vi "Distance and Turn Conversion.vi"(6 "Turn?":bool, 8 "Inches/Degrees Left":dbl, 9 "CAN Talon SRX Ref Left In":T1={"DeviceStatus"={"status"=FALSE, "code"=0, "source"=""}, "Type"=enum."PWM", "PWM"={"PWM Channel"=enum."PWM 1", "DeadBand"={"Name"="", "maxPositivePwm"=0, "minPositivePwm"=0, "centerPwm"=0, "maxNegativePwm"=0, "minNegativePwm"=0, "angularRange"=0}}, "CAN"={"Device Number"=0, "SetOutput VI Ref"=variant(enum8{"Percent VBus", "Current", "Speed", "Position", "Voltage"} enum."Percent VBus"), "GetOutput VI Ref"=variant(refnum<k1> refnum), "Enable VI Ref"=variant(dbl 12.0), "Disable VI Ref"=variant(enum8{"Percent VBus", "Speed", "Position", "Slave", "Unchanged / Invalid", "Voltage Compensation", "Current", "Motion Profile"} enum."Percent VBus"), "Data"=variant}, "Invert"=FALSE}, 10 "Inches/Degrees Right":dbl, 11 "CAN Talon SRX Ref Right In":T1={"DeviceStatus"={"status"=FALSE, "code"=0, "source"=""}, "Type"=enum."PWM", "PWM"={"PWM Channel"=enum."PWM 1", "DeadBand"={"Name"="", "maxPositivePwm"=0, "minPositivePwm"=0, "centerPwm"=0, "maxNegativePwm"=0, "minNegativePwm"=0, "angularRange"=0}}, "CAN"={"Device Number"=0, "SetOutput VI Ref"=variant(enum8{"Percent VBus", "Current", "Speed", "Position", "Voltage"} enum."Percent VBus"), "GetOutput VI Ref"=variant(refnum<k1> refnum), "Enable VI Ref"=variant(dbl 12.0), "Disable VI Ref"=variant(enum8{"Percent VBus", "Speed", "Position", "Slave", "Unchanged / Invalid", "Voltage Compensation", "Current", "Motion Profile"} enum."Percent VBus"), "Data"=variant}, "Invert"=FALSE}) -> (1 "CAN Talon SRX Ref Left Out":T1={"DeviceStatus"={"status"=FALSE, "code"=0, "source"=""}, "Type"=enum."PWM", "PWM"={"PWM Channel"=enum."Invalid", "DeadBand"={"Name"="", "maxPositivePwm"=0, "minPositivePwm"=0, "centerPwm"=0, "maxNegativePwm"=0, "minNegativePwm"=0, "angularRange"=0}}, "CAN"={"Device Number"=0, "SetOutput VI Ref"=variant, "GetOutput VI Ref"=variant, "Enable VI Ref"=variant, "Disable VI Ref"=variant, "Data"=variant}, "Invert"=FALSE}, 3 "CAN Talon SRX Ref Right Out":T1={"DeviceStatus"={"status"=FALSE, "code"=0, "source"=""}, "Type"=enum."PWM", "PWM"={"PWM Channel"=enum."Invalid", "DeadBand"={"Name"="", "maxPositivePwm"=0, "minPositivePwm"=0, "centerPwm"=0, "maxNegativePwm"=0, "minNegativePwm"=0, "angularRange"=0}}, "CAN"={"Device Number"=0, "SetOutput VI Ref"=variant, "GetOutput VI Ref"=variant, "Enable VI Ref"=variant, "Disable VI Ref"=variant, "Data"=variant}, "Invert"=FALSE}, 4 "Both In Range":bool)   [LabVIEW 2016]
uses:
  <vilib>/Rock Robotics/WPI/MotorControl/WPI_MotorControlDeviceRef.ctl
  <vilib>/Rock Robotics/WPI/MotorControl/WPI_MotorControlType.ctl
  <vilib>/Rock Robotics/SystemInterfaces/DIO/FPGA_DIOPWMChannel.ctl
  <vilib>/Rock Robotics/WPI/PWM/WPI_PWMDeadband.ctl
  <vilib>/Rock Robotics/WPI/ThirdParty/CanMotor/TalonSRX/WPI_CANTalonSRX_APIControlMode.ctl
panel:
  out "Right Rotations":dbl
  out "Left Rotations":dbl
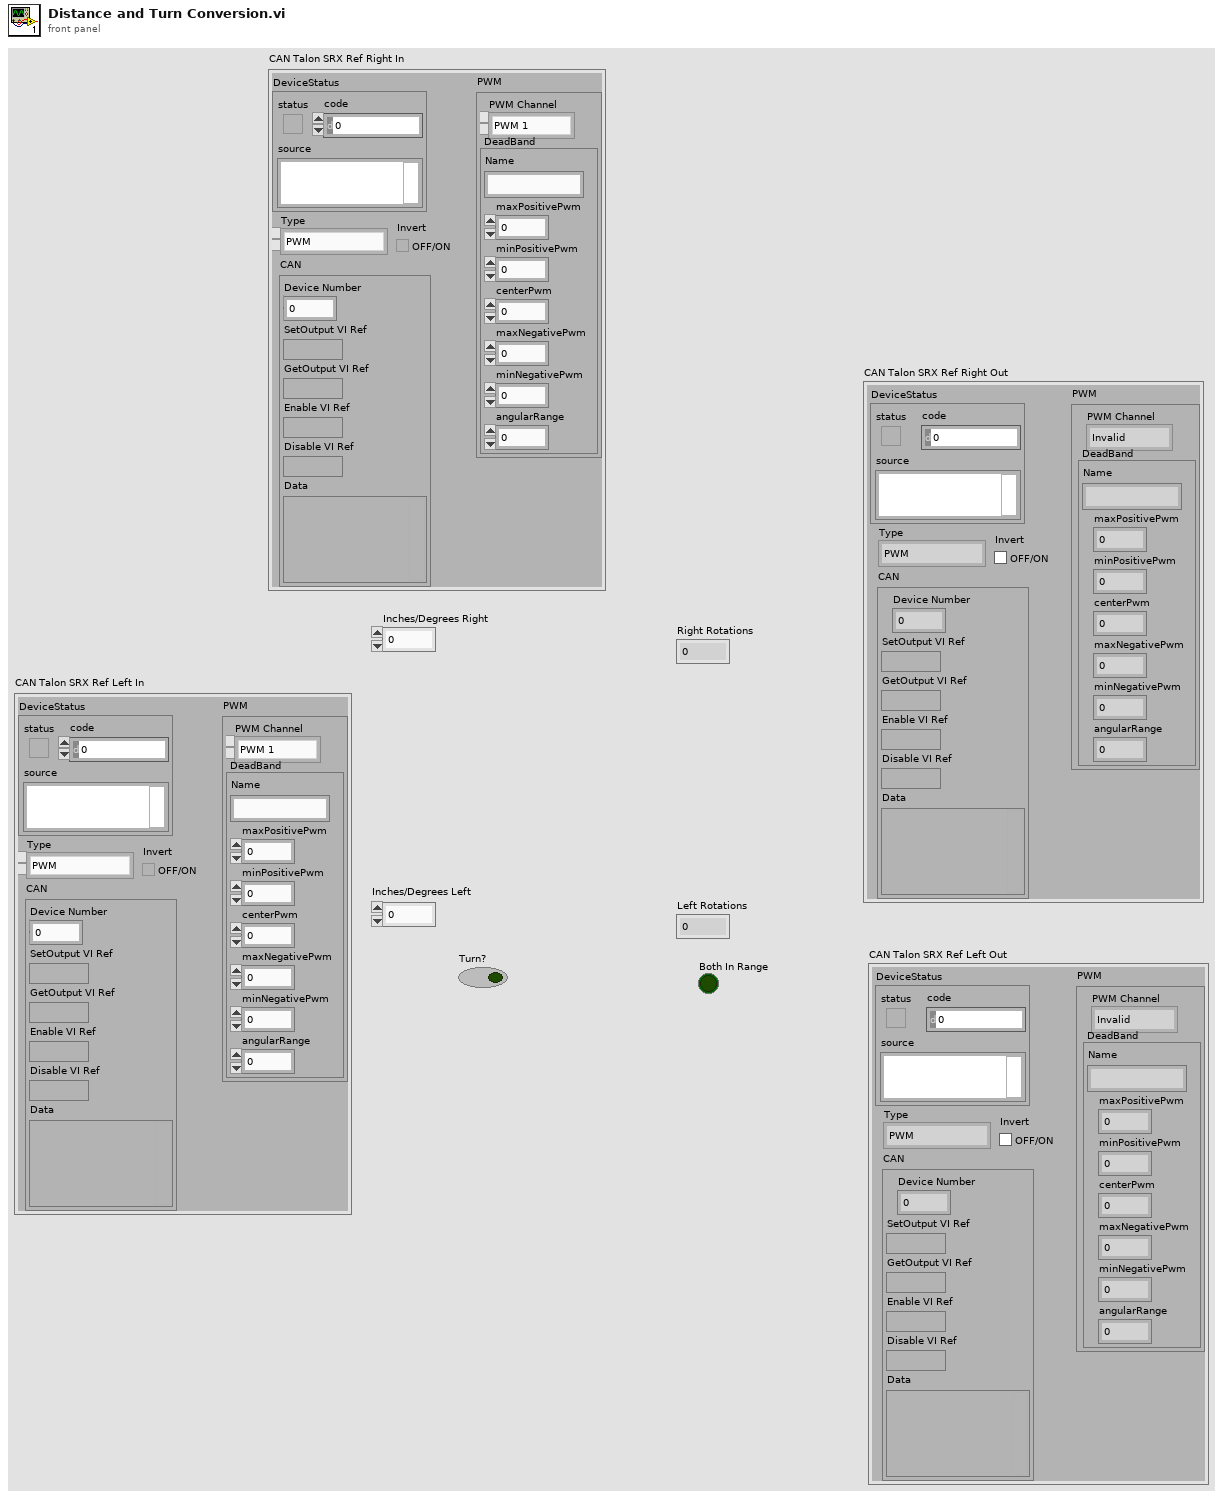
[diagram p1: front panel]
types:
  T1 = typedef "WPI_MotorControlDeviceRef.ctl" = cluster{"DeviceStatus":errorcluster, "Type":T2, "PWM":cluster{"PWM Channel":T3, "DeadBand":T4}, "CAN":cluster{"Device Number":u8, "SetOutput VI Ref":variant, "GetOutput VI Ref":variant, "Enable VI Ref":variant, "Disable VI Ref":variant, "Data":variant}, "Invert":bool}
  T2 = typedef "WPI_MotorControlType.ctl" = enum16{"PWM", "CAN"}
  T3 = typedef "FPGA_DIOPWMChannel.ctl" = enum8{"PWM 0", "PWM 1", "PWM 2", "PWM 3", "PWM 4", "PWM 5", "PWM 6", "PWM 7", "PWM 8", "PWM 9", "PWM MXP 0", "PWM MXP 1", "PWM MXP 2", "PWM MXP 3", "PWM MXP 4", "PWM MXP 5", "PWM MXP 6", "PWM MXP 7", "PWM MXP 8", "PWM MXP 9", "Invalid"}
  T4 = typedef "WPI_PWMDeadband.ctl" = cluster{"Name":string, "maxPositivePwm":i32, "minPositivePwm":i32, "centerPwm":i32, "maxNegativePwm":i32, "minNegativePwm":i32, "angularRange":u16}
  T5 = typedef "WPI_CANTalonSRX_APIControlMode.ctl" = enum8{"Percent VBus", "Speed", "Position", "Slave", "Unchanged / Invalid", "Voltage Compensation", "Current", "Motion Profile", "Motion Magic"}
  T6 = typedef "WPI_CANTalonSRX_GlobalStatus.ctl" = cluster{"Applied Throttle":dbl, "Module Enabled":bool, "CAN Error":errorcluster, "Closed Loop Error":dbl, "Forward Limit Switch Closed":bool, "Reverse Limit Switch Closed":bool, "Sensor Position":dbl, "Sensor Velocity":dbl, "Current":dbl, "Sticky Fault - Over Temp":bool, "Sticky Fault - Under Voltage":bool, "Sticky Fault - Forward Limit":bool, "Sticky Fault - Reverse Limit":bool, "Sticky Fault - Forward Soft Limit":bool, "Sticky Fault - Reverse Soft Limit":bool, "Brake is Enabled":bool, "Encoder Position":dbl, "Encoder Velocity":dbl, "Encoder Index Count":dbl, "Encoder A Pin State":bool, "Encoder B Pin State":bool, "Encoder Index Pin State":bool, "Analog In":dbl, "Analog In Velocity":dbl, "Temperature (C)":dbl, "Battery Voltage":dbl, "Control 5 Is Supported":bool, "Current Profile Slot Select":dbl, "Pos Div 8":bool, "Vel Div 4":bool, "Pulse Width Position":i32, "Pulse Width Velocity":i32, "Pulse Width Rise To Rise (us)":i32, "Pulse Width Rise To Fall (us)":i32, "Mot Prof Active Is Under Run":bool, "Mot Prof Active Has Under Run":bool, "Mot Prof Active Is Last":bool, "Mot Prof Active Velocity Only":bool, "Mot Prof Active Is Valid":bool, "Mot Prof Buffer Is Full":bool, "Mot Prof Active Profile Slot Select":i32, "Mot Prof NextID":i32, "Mot Prof Count":i32, "Mot Prof Active Velocity":dbl, "Mot Prof Active Position":dbl, "Mot Prof Output Enable":i32}
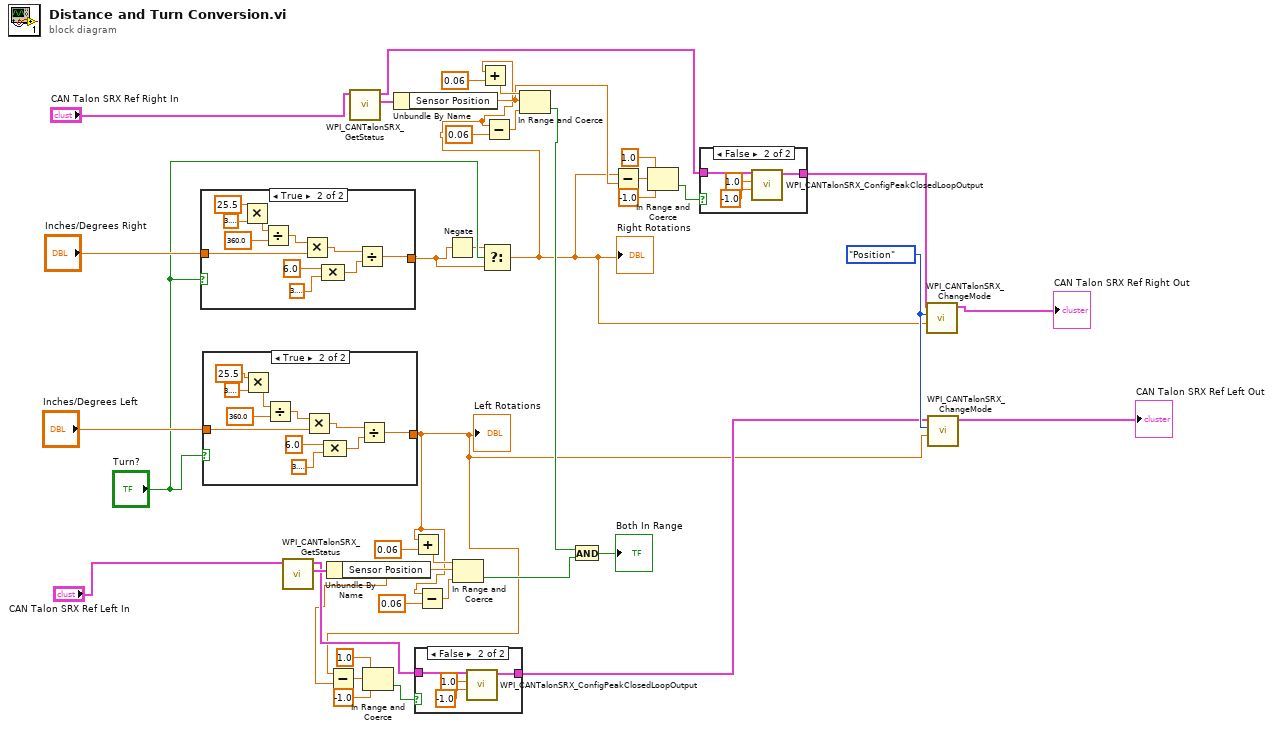
[diagram p0: block diagram]
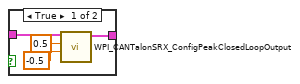
[diagram p2: hidden frame]
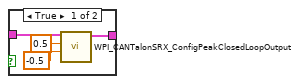
[diagram p3: hidden frame]
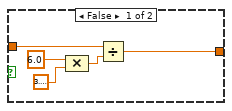
[diagram p4: hidden frame]
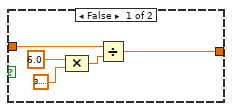
[diagram p5: hidden frame]
diagram:
  w7 = WPI_CANTalonSRX_APIControlMode."Position" ("Control Mode")
  n1 = case shown="True" "Turn?" {
    tunnel: "Inches/Degrees Right" -> [w42 w53]
    tunnel: [w40 w48] -> w35
    frame False {
      n2 = Compound Arithmetic op=MULTIPLY(6.0 ("value"), 3.141592653589793) -> (w41:dbl)
      n3 = Divide(x=w42, y=w41) -> (x/y=w40:dbl)
    }
    frame True {
      n4 = Multiply(x=25.5, y=3.141592653589793) -> (x*y=w46:dbl)
      n5 = Divide(x=w46, y=360.0) -> (x/y=w54:dbl)
      n6 = Multiply(x=w54, y=w53) -> (x*y=w49:dbl)
      n7 = Compound Arithmetic op=MULTIPLY(6.0 ("value"), 3.141592653589793) -> (w50:dbl)
      n8 = Divide(x=w49, y=w50) -> (x/y=w48:dbl)
    }
  }
  n9 = case shown="True" "Turn?" {
    tunnel: "Inches/Degrees Left" -> [w58 w69]
    tunnel: [w56 w64] -> w1
    frame False {
      n10 = Compound Arithmetic op=MULTIPLY(6.0 ("value"), 3.141592653589793) -> (w57:dbl)
      n11 = Divide(x=w58, y=w57) -> (x/y=w56:dbl)
    }
    frame True {
      n12 = Multiply(x=25.5, y=3.141592653589793) -> (x*y=w62:dbl)
      n13 = Divide(x=w62, y=360.0) -> (x/y=w70:dbl)
      n14 = Multiply(x=w70, y=w69) -> (x*y=w65:dbl)
      n15 = Compound Arithmetic op=MULTIPLY(6.0 ("value"), 3.141592653589793) -> (w66:dbl)
      n16 = Divide(x=w65, y=w66) -> (x/y=w64:dbl)
    }
  }
  "Left Rotations" <- w1
  n17 = call <vilib>:"WPI_CANTalonSRX_GetStatus.vi"("CAN Talon SRX Ref"="CAN Talon SRX Ref Left In") -> ("Talon SRX Status"=w28:T6, "CAN Talon SRX Ref"=w15:T1)  [unwired: 8 in, 1 out]
  n18 = Unbundle By Name(w28) -> ("Sensor Position"=w14:dbl)
  n19 = Subtract(x=w1, y=w14) -> (x-y=w19:dbl)
  n20 = call <vilib>:"WPI_CANTalonSRX_GetStatus.vi"("CAN Talon SRX Ref"="CAN Talon SRX Ref Right In") -> ("Talon SRX Status"=w34:T6, "CAN Talon SRX Ref"=w8:T1)  [unwired: 8 in, 1 out]
  n21 = In Range and Coerce(upper limit=1.0, x=w19, lower limit=-1.0) -> (In Range?=w16:bool)  [unwired: 1 out]
  n22 = Unbundle By Name(w34) -> ("Sensor Position"=w9:dbl)
  n23 = Add(x=w1, y=0.06) -> (x+y=w27:dbl)
  n24 = case shown="False" w16 {
    tunnel: w15 -> [w75 w79]
    tunnel: [w74 w78] -> w5
    frame True {
      n25 = call <vilib>:"WPI_CANTalonSRX_ConfigPeakClosedLoopOutput.vi"("Reverse Peak Output"=-0.5, "Forward Peak Output"=0.5, "CAN Talon SRX Ref"=w75) -> ("CAN Talon SRX Ref"=w74:T1)  [unwired: 7 in, 1 out]
    }
    frame False {
      n26 = call <vilib>:"WPI_CANTalonSRX_ConfigPeakClosedLoopOutput.vi"("Reverse Peak Output"=-1.0, "Forward Peak Output"=1.0, "CAN Talon SRX Ref"=w79) -> ("CAN Talon SRX Ref"=w78:T1)  [unwired: 7 in, 1 out]
    }
  }
  n27 = Subtract(x=w1, y=0.06) -> (x-y=w25:dbl)
  n28 = Negate(x=w35) -> (-x=w36:dbl)
  n29 = In Range and Coerce(upper limit=w27, x=w14, lower limit=w25) -> (In Range?=w21:bool)  [unwired: 1 out]
  n30 = Select(t=w36, s="Turn?", f=w35) -> (s? t:f=w2:dbl)
  "Right Rotations" <- w2
  n31 = Add(x=w2, y=0.06) -> (x+y=w33:dbl)
  n32 = Subtract(x=w2, y=0.06) -> (x-y=w31:dbl)
  n33 = In Range and Coerce(upper limit=w33, x=w9, lower limit=w31) -> (In Range?=w22:bool)  [unwired: 1 out]
  n34 = And(x=w22, y=w21) -> (x .and. y?=→"Both In Range":bool)
  n35 = Subtract(x=w2, y=w9) -> (x-y=w13:dbl)
  n36 = In Range and Coerce(upper limit=1.0, x=w13, lower limit=-1.0) -> (In Range?=w10:bool)  [unwired: 1 out]
  n37 = case shown="False" w10 {
    tunnel: w8 -> [w83 w87]
    tunnel: [w82 w86] -> w6
    frame True {
      n38 = call <vilib>:"WPI_CANTalonSRX_ConfigPeakClosedLoopOutput.vi"("Reverse Peak Output"=-0.5, "Forward Peak Output"=0.5, "CAN Talon SRX Ref"=w83) -> ("CAN Talon SRX Ref"=w82:T1)  [unwired: 7 in, 1 out]
    }
    frame False {
      n39 = call <vilib>:"WPI_CANTalonSRX_ConfigPeakClosedLoopOutput.vi"("Reverse Peak Output"=-1.0, "Forward Peak Output"=1.0, "CAN Talon SRX Ref"=w87) -> ("CAN Talon SRX Ref"=w86:T1)  [unwired: 7 in, 1 out]
    }
  }
  n40 = call <vilib>:"WPI_CANTalonSRX_ChangeMode.vi"("Output"=w2, "Control Mode"=w7, "CAN Talon SRX Ref"=w6) -> ("CAN Talon SRX Ref"=→"CAN Talon SRX Ref Right Out":T1)  [unwired: 7 in, 1 out]
  n41 = call <vilib>:"WPI_CANTalonSRX_ChangeMode.vi"("Output"=w1, "Control Mode"=w7, "CAN Talon SRX Ref"=w5) -> ("CAN Talon SRX Ref"=→"CAN Talon SRX Ref Left Out":T1)  [unwired: 7 in, 1 out]
